vi "Esophageal_FastHRME_ColorCamera_Initialize.vi"(8 "error in (no error)":errorcluster) -> (0 "error out":errorcluster, 2 "HRME Image Reference":T2, 3 "OMS Camera Reference Out":T1 caption="FastHRME Camera Session Out")   [LabVIEW 2021]
uses:
  <vilib>/vision/Image Controls.llb/IMAQ Image.ctl
  <vilib>/userdefined/High Color/IMAQdx.ctl
  <vilib>/vision/driver/IMAQdx.llb/IMAQdx Acquisition Mode.ctl
  <vilib>/vision/driver/NI_Vision_Acquisition_Software.lvlib
  <resource>/objmgr/imaqdx.rc
panel:
  # "SubVI Inputs"
  # "SubVI Outputs"
  # "Mono"
  # "17301505"
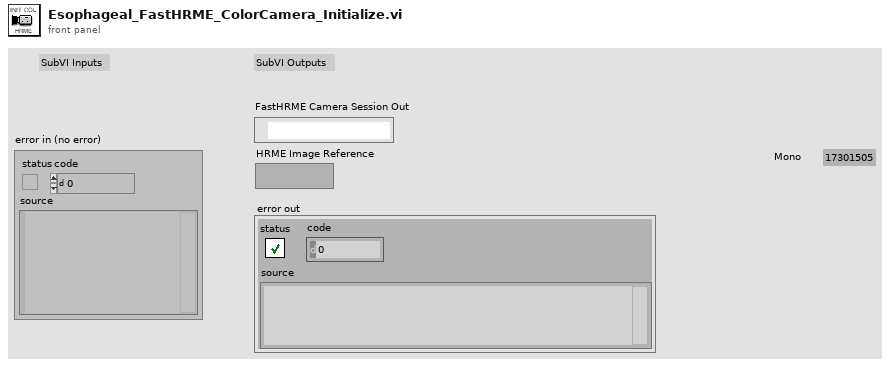
[diagram p1: front panel]
types:
  T1 = typedef "IMAQdx.ctl" = refnum<k21>
  T2 = typedef "IMAQ Image.ctl" = refnum<image>
  T3 = typedef "NI_Vision_Acquisition_Software.lvlib/IMAQdx Acquisition Mode.ctl" = enum32{"One Shot", "Continuous"}
  T4 = typedef "Image Type" = u32
  T5 = cluster{"Type":u32, "Version":u32, "Flags":u32, "SerialNumberHigh":u32, "SerialNumberLow":u32, "BusType":u32, "InterfaceName":string, "VendorName":string, "ModelName":string, "CameraFileName":string, "CameraAttributeURL":string}[]
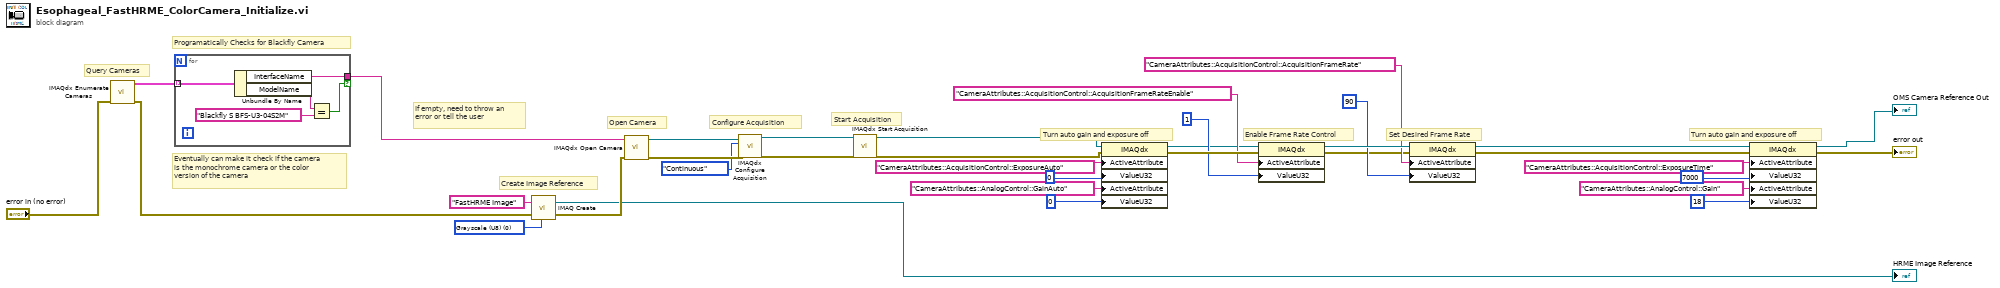
[diagram p0: block diagram]
diagram:
  w34 = T4 0 items=["Grayscale (U8)", "Grayscale (I16)", "Grayscale (SGL)", "Complex (CSG)", "RGB (U32)", "HSL (U32)", "RGB (U64)", "Grayscale (U16)"] ("Image Type")
  # "Turn auto gain and exposure off"
  # "Set Desired Frame Rate"
  # "Enable Frame Rate Control"
  # "Eventually can make it check if the camera\nis the monochrome camera or the color\nversion of the camera"
  # "If empty, need to throw an error or tell the user"
  # "Query Cameras"
  # "Programatically Checks for Blackfly Camera"
  # "Turn auto gain and exposure off"
  # "Start Acquisition"
  # "Configure Acquisition"
  # "Open Camera"
  # "Create Image Reference"
  n1 = call <vilib>:"IMAQdx Enumerate Cameras.vi"("error in"="error in (no error)") -> ("error out"=w9:errorcluster, "Camera Information Array"=w12:T5)  [unwired: 9 in]
  n2 = for {
    tunnel: w12 -> [w40] mode=indexing
    tunnel: [w37] -> w11 if=w36
    n3 = Unbundle By Name(w40) -> ("InterfaceName"=w37:string, "ModelName"=w39:string)
    n4 = Equal?(x=w39, y="Blackfly S BFS-U3-04S2M") -> (x = y?=w36:bool)
  }
  n5 = call "IMAQ Create"("Image Name"="FastHRME Image", "Image Type"=w34, "error in (no error)"=w9) -> ("New Image"=→"HRME Image Reference":T2, "error out"=w28:errorcluster)  [unwired: 2 in]
  n6 = call <vilib>:"IMAQdx Open Camera.vi"("error in"=w28, "Session In"=w11) -> ("error out"=w32:errorcluster, "Session Out"=w33:T1)  [unwired: 8 in]
  n7 = call <vilib>:"IMAQdx Configure Acquisition.vi"("error in"=w32, "Continuous?"=IMAQdx_Acquisition_Mode."Continuous", "Session In"=w33) -> ("error out"=w29:errorcluster, "Session Out"=w30:T1)  [unwired: 7 in]
  n8 = call <vilib>:"IMAQdx Start Acquisition.vi"("error in"=w29, "Session In"=w30) -> ("error out"=w22:errorcluster, "Session Out"=w21:T1)  [unwired: 8 in]
  n9 = property class="IMAQdx"(reference=w21, error in=w22, "ActiveAttribute"="CameraAttributes::AcquisitionControl::ExposureAuto", "ValueU32"=u32 0, "ActiveAttribute"="CameraAttributes::AnalogControl::GainAuto", "ValueU32"=u32 0) -> (reference out=w13:T1, error out=w20:errorcluster)
  n10 = property class="IMAQdx"(reference=w13, error in=w20, "ActiveAttribute"="CameraAttributes::AcquisitionControl::AcquisitionFrameRateEnable", "ValueU32"=u32 1) -> (reference out=w19:T1, error out=w14:errorcluster)
  n11 = property class="IMAQdx"(reference=w19, error in=w14, "ActiveAttribute"="CameraAttributes::AcquisitionControl::AcquisitionFrameRate", "ValueU32"=u32 90) -> (reference out=w1:T1, error out=w4:errorcluster)
  n12 = property class="IMAQdx"(reference=w1, error in=w4, "ActiveAttribute"="CameraAttributes::AcquisitionControl::ExposureTime", "ValueU32"=u32 7000, "ActiveAttribute"="CameraAttributes::AnalogControl::Gain", "ValueU32"=u32 18) -> (reference out=→"OMS Camera Reference Out":T1, error out=→"error out":errorcluster)
